vi "Global variable template.vi"() -> ()   [LabVIEW 2021]
uses:
  Globals and TypeDefs/Type Definitions.llb/McPherson Grating Density.ctl
  Globals and TypeDefs/Type Definitions.llb/Wavelength Unit.ctt
  Globals and TypeDefs/Type Definitions.llb/3 way Status.ctl
  Globals and TypeDefs/Error Categories.ctt
  <vilib>/Utility/error.llb/DialogType.ctl
  Globals and TypeDefs/gDetector.vi
  Globals and TypeDefs/gGeneral.vi
  Globals and TypeDefs/gHField.vi
  Globals and TypeDefs/gSpectrometer.vi
  Globals and TypeDefs/gStatus.vi
  Globals and TypeDefs/gTemperature.vi
panel:
  in  "Case Constant\n(See Context Help)":bool
  in  "Wavelength Unit":T1
  in  "Grating Density (g/mm)":T2=enum."1200" caption="Grating Density"
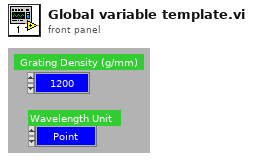
[diagram p1: front panel]
types:
  T1 = typedef "Wavelength Unit.ctt" = enum8{"Point", "nm", "eV", "meV", "cm_1"}
  T2 = typedef "McPherson Grating Density.ctl" = enum8{"150", "300", "600", "1200", "1800"}
  T3 = typedef "3 way Status.ctl" = u8
  T4 = enum8{"Initialization Error", "Command Error", "Parameter Error", "Overflow Error", "Time-out Error", "Misc Error", "User cancel"}
  T5 = typedef "Error Categories.ctt" = enum8{"General", "CCD-256x1024", "CCD-1340x400", "InGaAs PDA", "McPherson 2075", "Magnetic Field", "Temperature Control", "Other"}
  T6 = typedef "DialogType.ctl" = u16
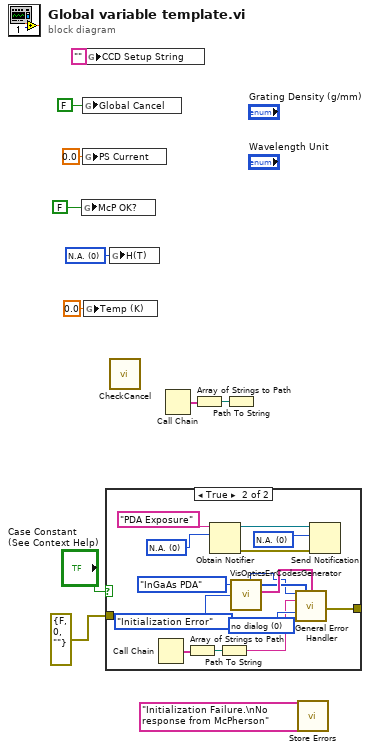
[diagram p0: block diagram]
diagram:
  w4 = T3 0 items=["N.A.", "OK", "Busy", "Done"] ("H(T)")
  n1 = global write "gSpectrometer.vi" "McP OK?"(FALSE ("McP OK?")) -> ()
  n2 = global write "gGeneral.vi" "Global Cancel"(FALSE ("Global Cancel")) -> ()
  n3 = global write "gHField.vi" "PS Current"(0.0 ("PS Current")) -> ()
  n4 = global write "gTemperature.vi" "Temp (K)"(0.0 ("Temp (K)")) -> ()
  n5 = global write "gDetector.vi" "CCD Setup String"("" ("CCD Setup String")) -> ()
  n6 = case shown="True" "Case Constant\n(See Context Help)" {
    tunnel: [w12 w22] -> _
    tunnel: errorcluster {"status"=FALSE, "code"=0, "source"=""} ("error out") -> [w12 _]
    frame False {
    }
    frame True {
      w13 = T3 0 items=["N.A.", "OK", "Busy", "Done"] ("notification")
      w17 = T3 0 items=["N.A.", "OK", "Busy", "Done"] ("Saving")
      w27 = T6 0 items=["no dialog", "OK message", "continue or stop message", "OK message + warnings", "continue/stop + warnings"] ("type of dialog (OK msg:1)")
      n7 = Call Chain() -> (call chain=w20:string[])
      n8 = Array of Strings to Path(0:w20) -> (2:w19:path)  [unwired: 1 in]
      n9 = Obtain Notifier(name (unnamed)="PDA Exposure", notification data type=w17) -> (notifier out=w15:refnum<notifier>, error out=w14:errorcluster)  [unwired: 2 in, 1 out]
      n10 = Path To String(path=w19) -> (string=w18:string)
      n11 = call "VisOpticsErrCodesGenerator.vi"("NHMFL Visible Optics Error Type"=T4."Initialization Error", "NHMFL Visible Optics Error Categories"=Error_Categories.ctt."InGaAs PDA") -> ("user-defined descriptions"=w26:string[], "User-defined Error Code"=w21:i32, "user-defined codes"=w25:i32[])  [unwired: 1 in, 3 out]
      n12 = call <vilib>:"General Error Handler.vi"("[error code] (0)"=w21, "[user-defined codes]"=w25, "[user-defined descriptions]"=w26, "[error source] (\" \")"=w18, "type of dialog (OK msg:1)"=w27) -> ("error out"=w22:errorcluster)  [unwired: 6 in, 4 out]
      n13 = Send Notification(notification=w13, notifier=w15, error in (no error)=w14) -> ()  [unwired: 2 out]
    }
  }
  n14 = global write "gStatus.vi" "H(T)"(w4) -> ()
  n15 = call "CheckCancel.vi"() -> ()  [unwired: 2 in, 2 out]
  n16 = Call Chain() -> (call chain=w11:string[])
  n17 = Array of Strings to Path(0:w11) -> (2:w10:path)  [unwired: 1 in]
  n18 = Path To String(path=w10) -> ()  [unwired: 1 out]
  n19 = call "Store Errors.vi"("New Error"="Initialization Failure.\nNo response from McPherson") -> ()  [unwired: 1 in]
